vi "Call Perform Action.vi"(8 "error in (no error)":errorcluster, 10 "Input":variant, 11 "Task Base in":refnum<class "Task Base.lvclass">) -> (0 "error out":errorcluster, 2 "Output":variant, 3 "Task Base out":refnum<class "Task Base.lvclass">)   [LabVIEW 2023, in "HAL GOOP4.lvlib" / "Task Base.lvclass"]
uses:
  Study Base/Study Base.lvclass/Study Base.ctl
  Task Base.lvclass
  Task Base.lvclass/Task Base.ctl
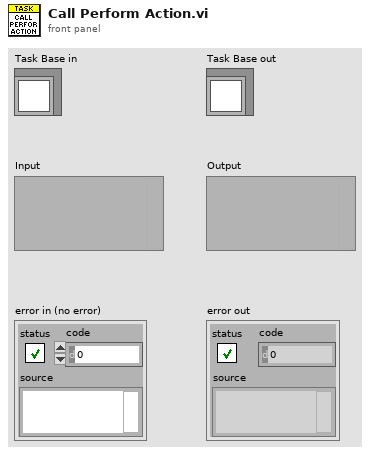
[diagram p1: front panel]
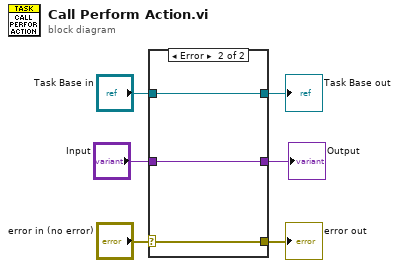
[diagram p0: block diagram]
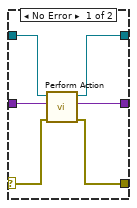
[diagram p2: hidden frame]
diagram:
  n1 = case shown="Error" "error in (no error)" {
    selector: "error in (no error)" -> [w9 w15]
    tunnel: [w8 w15] -> w5
    tunnel: [w11 w14] -> w3
    tunnel: "Task Base in" -> [w12 w14]
    tunnel: "Input" -> [w10 w13]
    tunnel: [w7 w13] -> w1
    frame No Error {
      n2 = call-dynamic "Perform Action.vi"("error in (no error)"=w9, "Input"=w10, "Task Base in"=w12) -> ("error out"=w8:errorcluster, "Output"=w7:variant, "Task Base out"=w11:refnum<class "Task Base.lvclass">)  [unwired: 6 in]
    }
    frame Error {
    }
  }
  "error out" <- w5
  "Task Base out" <- w3
  "Output" <- w1
